vi "ChannelSettings.vi"(8 "Channel_Enum":T1=1 items=["4-20_OUT", "Pres_HI1", "Pres_HI2", "Pres_LOW", "Pres_PIN", "HEATER_TOP", "HEATER_BOT", "T_Shell", "FLOWMETER", "WATT_SENSE", "WH_TICK", "Tc_1", "Tc_2", "Tc_3", "Tc_4", "Tc_5", "Tc_6", "Tc_down", "T_Shell_2", "T_Shell_3", "T_Shell_4", "RTD_IN", "RTD_OUT", "RTD_AMB", "INTF_TEMPFLO", "INTF_READY", "INTF_START", "INTF_STOP", "DRM_LOW", "DRM_HIGH", "PWR_MAIN", "VLV_DUMP", "VLV_OUT", "VLV_IN", "WATT_HOURS", "FLOW(SAMPLE)", "GALLONS", "FLOW(GPM)", "FLOW_CALC_GAIN", "FLOW_CALC_OFFSET", "FLOW_CALC_THRESHOLD", "VLV_DUMP_2", "VLV_OUT_2", "VLV_IN_2", "VLV_DUMP_3", "VLV_OUT_3", "VLV_IN_3", "VLV_DUMP_4", "VLV_OUT_4", "VLV_IN_4", "CHAN_34", "CHAN_35", "CHAN_36"]) -> (0 "Channel String":string)   [LabVIEW 2014]
uses:
  ChannelSettings.ctl
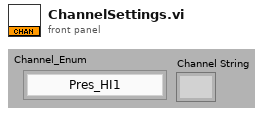
[diagram p1: front panel]
types:
  T1 = typedef "ChannelSettings.ctl" = u32
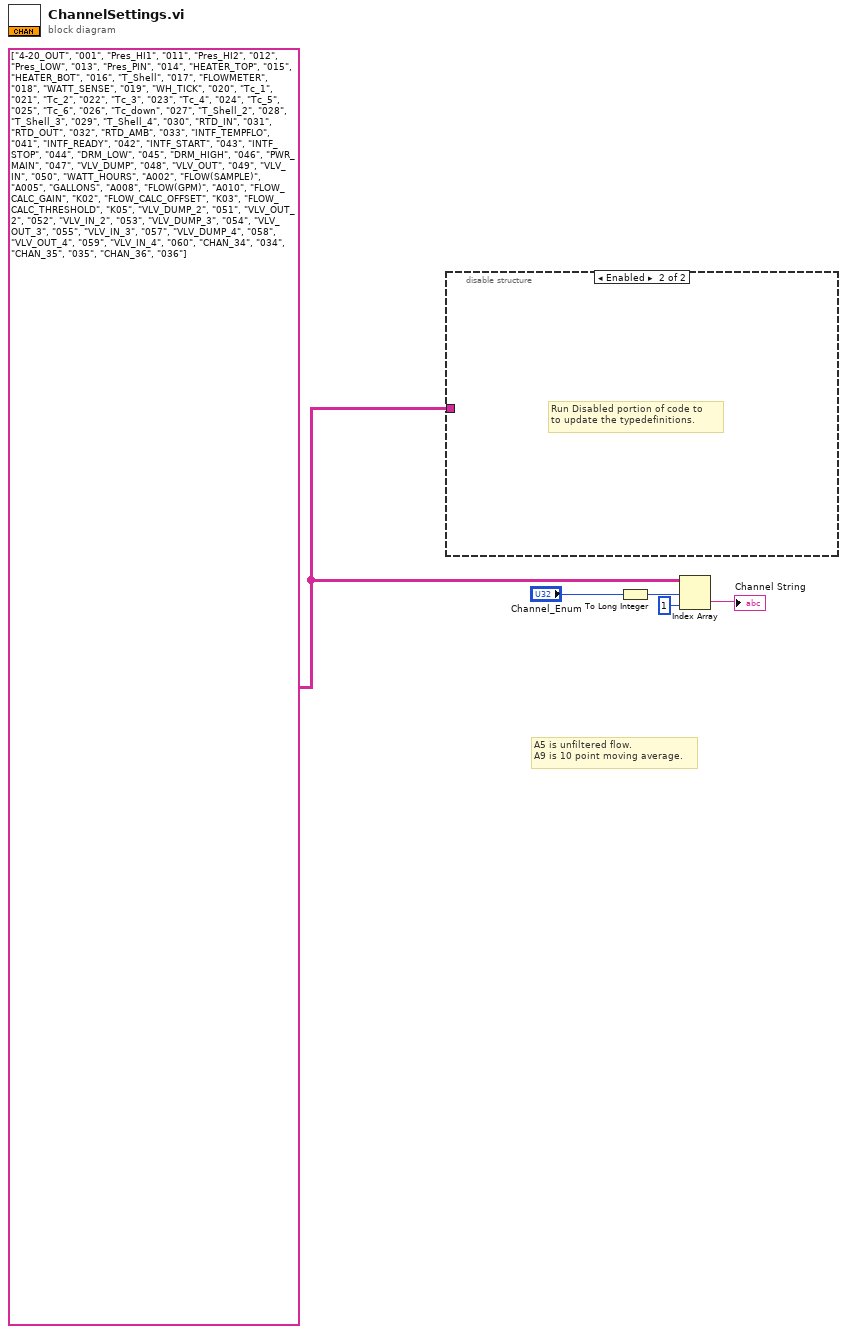
[diagram p0: block diagram]
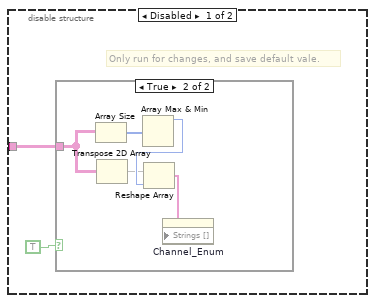
[diagram p2: hidden frame]
diagram:
  w2 = string[][] [["4-20_OUT", "001"], ["Pres_HI1", "011"], ["Pres_HI2", "012"], ["Pres_LOW", "013"], ["Pres_PIN", "014"], ["HEATER_TOP", "015"], ["HEATER_BOT", "016"], ["T_Shell", "017"], ["FLOWMETER", "018"], ["WATT_SENSE", "019"], ["WH_TICK", "020"], ["Tc_1", "021"], ["Tc_2", "022"], ["Tc_3", "023"], ["Tc_4", "024"], ["Tc_5", "025"], ["Tc_6", "026"], ["Tc_down", "027"], ["T_Shell_2", "028"], ["T_Shell_3", "029"], ["T_Shell_4", "030"], ["RTD_IN", "031"], ["RTD_OUT", "032"], ["RTD_AMB", "033"], ["INTF_TEMPFLO", "041"], ["INTF_READY", "042"], ["INTF_START", "043"], ["INTF_STOP", "044"], ["DRM_LOW", "045"], ["DRM_HIGH", "046"], ["PWR_MAIN", "047"], ["VLV_DUMP", "048"], ["VLV_OUT", "049"], ["VLV_IN", "050"], ["WATT_HOURS", "A002"], ["FLOW(SAMPLE)", "A005"], ["GALLONS", "A008"], ["FLOW(GPM)", "A010"], ["FLOW_CALC_GAIN", "K02"], ["FLOW_CALC_OFFSET", "K03"], ["FLOW_CALC_THRESHOLD", "K05"], ["VLV_DUMP_2", "051"], ["VLV_OUT_2", "052"], ["VLV_IN_2", "053"], ["VLV_DUMP_3", "054"], ["VLV_OUT_3", "055"], ["VLV_IN_3", "057"], ["VLV_DUMP_4", "058"], ["VLV_OUT_4", "059"], ["VLV_IN_4", "060"], ["CHAN_34", "034"], ["CHAN_35", "035"], ["CHAN_36", "036"]] ("Sorted 2D Array")
  # "A5 is unfiltered flow.\nA9 is 10 point moving average."
  n1 = disable-structure shown="Enabled" {
    disable-tunnel: w2 -> [w6 _]
    frame Disabled {
      # "Only run for changes, and save default vale."
      n2 = case shown="True" TRUE {
        tunnel: w6 -> [_ w10]
        frame False {
        }
        frame True {
          n3 = Array Size(array=w10) -> (size(s)=w12:i32[])
          n4 = Transpose 2D Array(2D array=w10) -> (transposed array=w9:string[][])
          n5 = Array Max & Min(array=w12) -> (max value=w11:i32)  [unwired: 3 out]
          n6 = Reshape Array(w9, w11) -> (w8:string[])
          n7 = property on="Channel_Enum" class="Ring (strict)"("Strings []"=w8) -> ()  [unwired: 2 in, 2 out]
        }
      }
    }
    frame Enabled {
      # "Run Disabled portion of code to \nto update the typedefinitions."
    }
  }
  n8 = To Long Integer(number="Channel_Enum") -> (32bit integer=w3:i32)
  n9 = Index Array(array=w2, index (row)=w3, index (col)=1 ("disabled index (col)")) -> (element=→"Channel String":string)
